vi "open mb.vi"(8 "error in (no error)":errorcluster) -> (0 "Error out":errorcluster)   [LabVIEW 2016, in "超标留样集成.lvlib" / "DR803M4.lvlib"]
uses:
  DR803M4.lvlib
  Global variable/hold variable.vi
  Global variable/input variable.vi
  <vilib>/Plasmionique/MB Master/MB_Master_Serial/MB_Master_Serial.lvclass
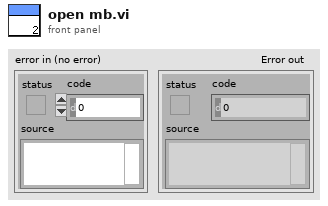
[diagram p1: front panel]
types:
  T1 = cluster{"baud rate (bps)":u32, "stop bits":u16, "parity":u16, "flow control":u16, "timeout":u32, "retries":i32}
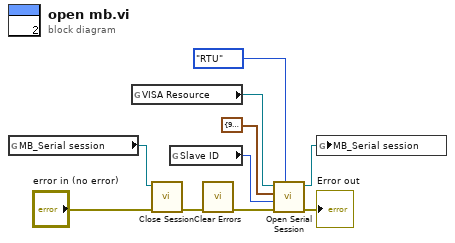
[diagram p0: block diagram]
diagram:
  n1 = global read "input variable.vi" "MB_Serial session"() -> (w3:refnum<class "MB_Master_Serial.lvclass">)
  n2 = global read "hold variable.vi" "VISA Resource"() -> (w7:refnum<visa-resource-name>)
  n3 = call-dynamic "Close Session.vi"("error in (no error)"="error in (no error)", "MB_Serial session"=w3) -> ("error out"=w10:errorcluster)  [unwired: 9 in]
  n4 = global read "hold variable.vi" "Slave ID"() -> (w8:u8)
  n5 = call <vilib>:"Clear Errors.vi"("error in (no error)"=w10) -> ("error out"=w9:errorcluster)  [unwired: 5 in, 1 out]
  n6 = call <vilib>:"Open Serial Session.vi"("Mode (RTU)"=enum16{"RTU", "ASCII"}."RTU", "Error in"=w9, "Slave ID"=w8, "Serial Config"=T1 {"baud rate (bps)"=9600, "stop bits"=10, "parity"=0, "flow control"=0, "timeout"=1000, "retries"=1}, "VISA Resource"=w7) -> ("Error out"=→"Error out":errorcluster, "MB_Serial session"=w2:refnum<class "MB_Master_Serial.lvclass">)  [unwired: 5 in]
  n7 = global write "input variable.vi" "MB_Serial session"(w2) -> ()
